vi "Write configuration.vi"(8 "error in":errorcluster, 10 "configuration":refnum<class "NISE_CEF_serializable configuration.lvclass">, 11 "PLTarget cRIO in":refnum<class "PLTarget cRIO.lvclass">) -> (0 "error out":errorcluster, 3 "PLTarget cRIO out":refnum<class "PLTarget cRIO.lvclass">)   [LabVIEW 2013, in "PLTarget cRIO.lvclass"]
uses:
  PLTarget cRIO.lvclass
  Framework Configuration Classes/target configuration/PL_Target Configuration.lvclass
  <vilib>/NI/CEF/CEF_TreeControl/serializable configuration/NISE_CEF_serializable configuration.lvclass
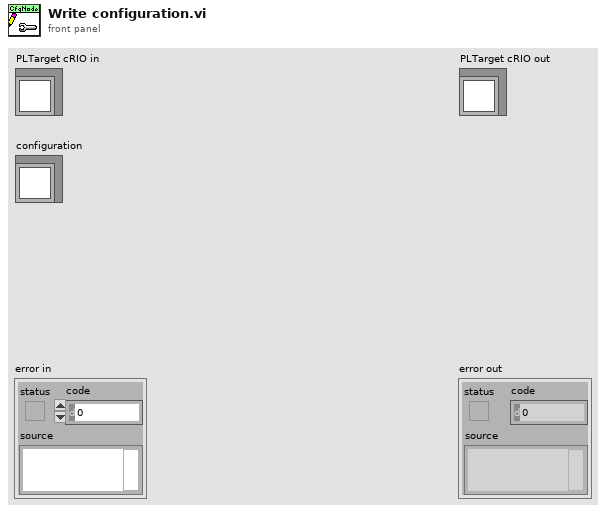
[diagram p1: front panel]
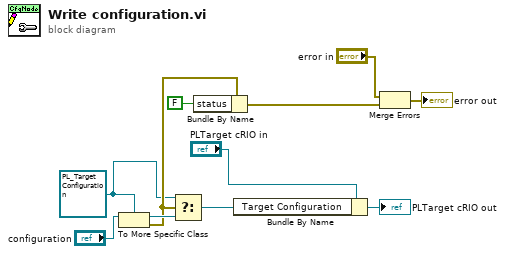
[diagram p0: block diagram]
diagram:
  w7 = refnum<class "PL_Target Configuration.lvclass"> refnum ("Target Configuration")
  n1 = To More Specific Class(target class=w7, reference="configuration") -> (specific class reference=w11:refnum<class "PL_Target Configuration.lvclass">, error out=w10:errorcluster)  [unwired: 1 in]
  n2 = Select(t=w7, s=w10, f=w11) -> (s? t:f=w6:refnum<class "PL_Target Configuration.lvclass">)
  n3 = Bundle By Name(cluster=w10, "status"=FALSE) -> (w8:errorcluster)
  n4 = Bundle By Name(cluster="PLTarget cRIO in", "Target Configuration"=w6) -> (→"PLTarget cRIO out":refnum<class "PLTarget cRIO.lvclass">)
  n5 = Merge Errors("error in", w8) -> (→"error out":errorcluster)
